vi "PH_PSDBWriter.constructor.vi"(0 "name":string, 2 "data in":string, 5 "error in":errorcluster) -> (14 "i ref out":refnum<vi>, 16 "data out":string, 19 "error out":errorcluster)   [LabVIEW 2014, in "PH_PSDBWriter.lvlib"]
doc: "This class is forseen to be inherited from. With its help data of devices can be stored in the PHELIX shot data base (PSDB). \n\n\n\nauthor: Stefan Götte, GSI\n\nLicense Agreement for this software:\n\nCopyright (C)\nGesellschaft für Schwerionenforschung, GSI\nPlanckstr. 1\n64291 Darmstadt\nGermany\n\nContact: D.Beck@gsi.de \n\nThis program is free software; you can redistribute it and/or modify it under the terms of the \nGNU General Public License as published by the Free Software Foundation; either version 2 of \nthe license, or (at your option) any later version.\n\nThis program is distributed in the hope that it will be useful, but WITHOUT ANY WARRANTY; \nwithout even the implied warranty of MERCHANTABILITY or FITNESS FOR A PARTICULAR PURPOSE. See the GNU General License for more details (http://www.gnu.org).\n\nGesellschaft für Schwerionenforschung, GSI\nPlanckstr. 1, 64291 Darmstadt, Germany\nFor all questions and ideas contact: M.Richter@gsi.de, H.Brand@gsi.de or D.Beck@gsi.de.\nLast update: 16-JUN-2004"
uses:
  PH_PSDBWriter.lvlib
  PH_PSDBWriter.Thread Commands.ctl
  PH_PSDBWriter.i attribute.ctl
  PH_PSDBWriter.PHELIX-Subsystems.ctl
  PH_PSDBWriter.Data Status.ctl
  PH_PSDBWriter.PSDB Dataset.ctl
  PH_PSDBWriter.2D dataset.ctl
  User/Eisenbarth/psdb_lv/PSDB_AxisDescription.ctl
  PH_PSDBWriter.Boolean dataset.ctl
  PH_PSDBWriter.Image dataset.ctl
  <vilib>/vision/Image Controls.llb/IMAQ Image.ctl
  PH_PSDBWriter.Numeric dataset.ctl
  PH_PSDBWriter.String dataset.ctl
  PH_Common/Connection/PH_Connection.PSDB Credentials.ctl
  CSCore/CSSystem/CSSystemLib/CSSystemLib.lvlib
  PH_Class/PH_Class.lvlib
  User/Eisenbarth/psdb_lv/PSDB.lvlib
  PH_Common/PH_Common.lvlib
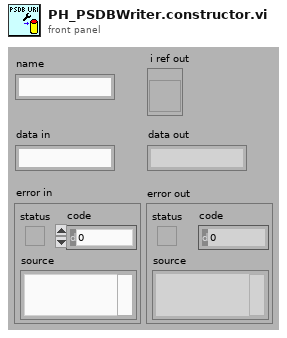
[diagram p1: front panel]
types:
  T1 = typedef "PH_PSDBWriter.lvlib/PH_PSDBWriter.i attribute.ctl" = cluster{"PSDB Status Service ID":i32, "Instance ID":i32, "Shot #":i32, "Subsystem":T2, "Data Status":T3, "Ref PSDB Status":refnum<vi>, "PSDB Error Code":i32, "PSDB Dataset":T4, "PSDB Thread":cluster{"Ref":refnum<vi>, "Q-Ref":refnum<queue>}, "PSDB Credentials":T12}
  T2 = typedef "PH_PSDBWriter.lvlib/PH_PSDBWriter.PHELIX-Subsystems.ctl" = i32
  T3 = typedef "PH_PSDBWriter.lvlib/PH_PSDBWriter.Data Status.ctl" = i16
  T4 = typedef "PH_PSDBWriter.lvlib/PH_PSDBWriter.PSDB Dataset.ctl" = cluster{"Version":i32, "2D data Input":T5[], "Boolean Input":T7[], "Image Input":T8[], "Numeric Input":T10[], "String Input":T11[]}
  T5 = typedef "PH_PSDBWriter.lvlib/PH_PSDBWriter.2D dataset.ctl" = cluster{"name":string, "data":dbl[][], "axis description":T6}
  T6 = typedef "PSDB.lvlib/PSDB_AxisDescription.ctl" = cluster{"x axis label":string, "y axis label":string, "x axis unit":string, "y axis unit":string}
  T7 = typedef "PH_PSDBWriter.lvlib/PH_PSDBWriter.Boolean dataset.ctl" = cluster{"name":string, "data":bool, "unit":string}
  T8 = typedef "PH_PSDBWriter.lvlib/PH_PSDBWriter.Image dataset.ctl" = cluster{"name":string, "data":T9, "unit":string}
  T9 = typedef "IMAQ Image.ctl" = refnum<image>
  T10 = typedef "PH_PSDBWriter.lvlib/PH_PSDBWriter.Numeric dataset.ctl" = cluster{"name":string, "data":dbl, "unit":string}
  T11 = typedef "PH_PSDBWriter.lvlib/PH_PSDBWriter.String dataset.ctl" = cluster{"name":string, "data":string, "unit":string}
  T12 = typedef "PH_Common.lvlib/PH_Connection.PSDB Credentials.ctl" = cluster{"PW":string, "ID":string, "DS":string}
  T13 = enum16{"SetAttribute", "GetAttribute", "CreateAttribute", "DestroyAttribute", "DestroyAllAtributes"}
  T14 = typedef "PH_PSDBWriter.lvlib/PH_PSDBWriter.Thread Commands.ctl" = u16
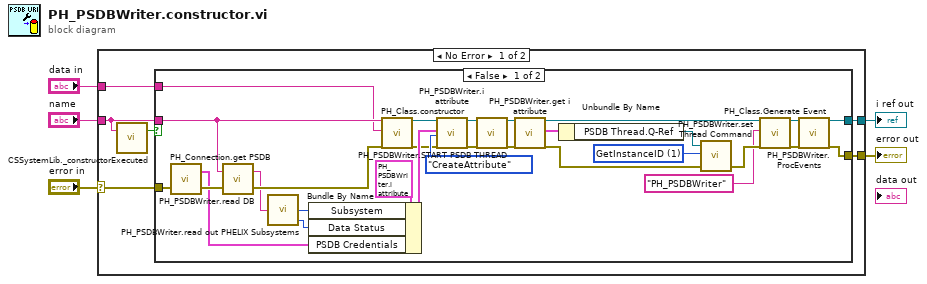
[diagram p0: block diagram]
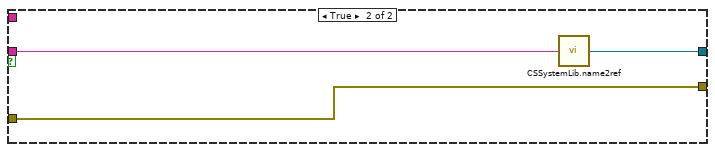
[diagram p2: hidden frame]
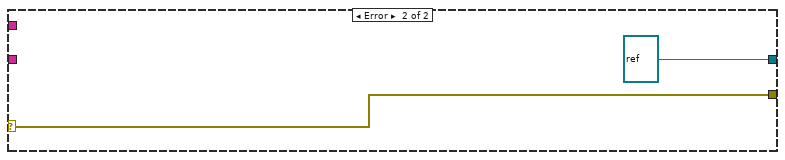
[diagram p3: hidden frame]
diagram:
  n1 = case shown="No Error" "error in" {
    selector: "error in" -> [w11 w45]
    tunnel: [w9 refnum<vi> refnum ("i ref out")] -> w5
    tunnel: [w10 w45] -> w4
    tunnel: "name" -> [w7 _]
    tunnel: "data in" -> [w8 _]
    frame No Error {
      n2 = call "CSSystemLib._constructorExecuted.vi"("name"=w7) -> ("constructor executed?"=w6:bool)  [unwired: 18 in]
      n3 = case shown="False" w6 {
        tunnel: w11 -> [w18 w41]
        tunnel: w7 -> [w19 w43]
        tunnel: [w37 w41] -> w10
        tunnel: [w36 w42] -> w9
        tunnel: w8 -> [w15 _]
        frame False {
          w33 = T14 1 items=["None", "GetInstanceID", "WriteToPSDB"] ("PSDB Thread Command")
          n4 = call "PH_Connection.get PSDB.vi"("error in (no error)"=w18) -> ("error out"=w13:errorcluster, "PSDB Credentials"=w12:T12)  [unwired: 1 in]
          n5 = call "PH_PSDBWriter.read DB.vi"("error in"=w13, "Instance Name"=w19) -> ("error out"=w17:errorcluster, "PSDB Subsystem"=w16:string)
          n6 = call "PH_PSDBWriter.read out PHELIX Subsystems.vi"("Config DB Subsystem"=w16) -> ("Metadata.Data Status"=w27:T3, "Metadata.Subsystem"=w28:T2)  [unwired: 2 in, 1 out]
          n7 = Bundle By Name(cluster=T1 {"PSDB Status Service ID"=-1, "Instance ID"=-1, "Shot #"=-1, "Subsystem"=-1, "Data Status"=-1, "Ref PSDB Status"=refnum, "PSDB Error Code"=0, "PSDB Dataset"={"Version"=0, "2D data Input"=[], "Boolean Input"=[], "Image Input"=[], "Numeric Input"=[], "String Input"=[]}, "PSDB Thread"={"Ref"=refnum, "Q-Ref"=refnum}, "PSDB Credentials"={"PW"="N/A", "ID"="N/A", "DS"="N/A"}} ("CLASS.i attribute"), "Subsystem"=w28, "Data Status"=w27, "PSDB Credentials"=w12) -> (w29:T1)
          n8 = call "PH_Class.constructor.vi"("name"=w19, "data in"=w15, "error in"=w17) -> ("i ref out"=w31:refnum<vi>, "error out"=w14:errorcluster)  [unwired: 14 in, 1 out]
          n9 = call "PH_PSDBWriter.i attribute.vi"("VI Refnum"=w31, "CLASS.i attribute"=w29, "Action"=T13."CreateAttribute", "error in (no error)"=w14) -> ("VI Refnum out"=w25:refnum<vi>, "error out"=w26:errorcluster)  [unwired: 13 in, 1 out]
          n10 = call "PH_PSDBWriter.START PSDB THREAD.vi"("VI in"=w25, "error in (no error)"=w26) -> ("VI out"=w39:refnum<vi>, "error out"=w32:errorcluster)  [unwired: 16 in]
          n11 = call "PH_PSDBWriter.get i attribute.vi"("i ref in"=w39, "error in (no error)"=w32) -> ("i ref out"=w24:refnum<vi>, "i attribute"=w35:T1, "error out"=w38:errorcluster)  [unwired: 15 in]
          n12 = Unbundle By Name(w35) -> ("PSDB Thread.Q-Ref"=w34:refnum<queue>)
          n13 = call "PH_PSDBWriter.set Thread Command.vi"("error in (no error)"=w38, "PSDB Thread Command"=w33, "Queue in"=w34) -> ("error out"=w22:errorcluster)  [unwired: 2 in]
          n14 = call "PH_Class.Generate Event.vi"("i ref in"=w24, "Class"="PH_PSDBWriter", "error in (no error)"=w22) -> ("i ref out"=w23:refnum<vi>, "error out"=w21:errorcluster)  [unwired: 15 in]
          n15 = call "PH_PSDBWriter.ProcEvents.vi"("i ref in"=w23, "error in"=w21) -> ("i ref out"=w36:refnum<vi>, "error out"=w37:errorcluster)  [unwired: 16 in]
        }
        frame True {
          n16 = call "CSSystemLib.name2ref.vi"("name"=w43) -> ("obj refnum"=w42:refnum<vi>)
        }
      }
    }
    frame Error {
    }
  }
  "i ref out" <- w5
  "error out" <- w4
